vi "Set Panel Origin.vi"(8 "error in (no error)":errorcluster, 10 "origin":T1, 11 "reference":refnum<vi>) -> (0 "error out":errorcluster)   [LabVIEW 2019, in "UI Tools.lvlib"]
doc: "Set origin of the Panel."
uses:
  UI Tools.lvlib
  <vilib>/Utility/miscctls.llb/LVPointTypeDef.ctl
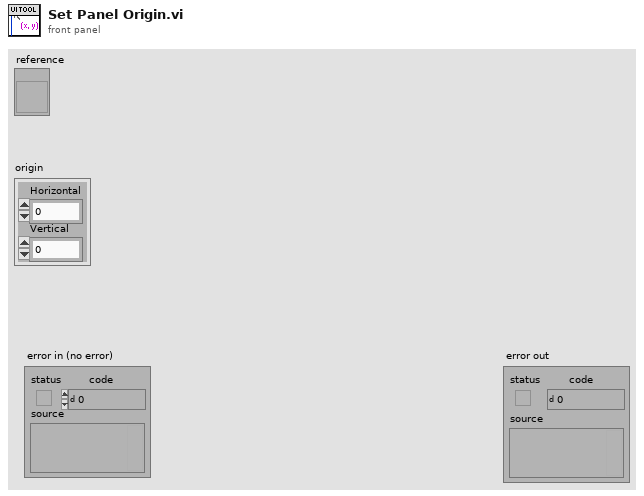
[diagram p1: front panel]
types:
  T1 = typedef "LVPointTypeDef.ctl" = cluster{"Horizontal":i16, "Vertical":i16}
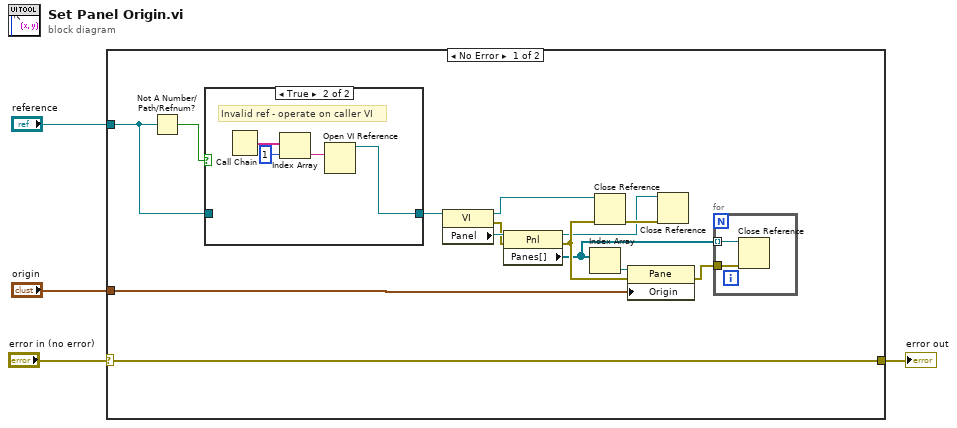
[diagram p0: block diagram]
diagram:
  n1 = case shown="No Error" "error in (no error)" {
    selector: "error in (no error)" -> [w18 w26]
    tunnel: [w18 w26] -> w3
    tunnel: "origin" -> [w5 _]
    tunnel: "reference" -> [w9 _]
    frame No Error {
      n2 = Not A Number/Path/Refnum?(number/path/refnum=w9) -> (NaN/Path/Refnum?=w10:bool)
      n3 = case shown="True" w10 {
        tunnel: [w19 w20] -> w8
        tunnel: w9 -> [w19 _]
        frame False {
        }
        frame True {
          # "Invalid ref - operate on caller VI"
          n4 = Call Chain() -> (call chain=w23:string[])
          n5 = Index Array(array=w23, index=1) -> (element=w21:string)
          n6 = Open VI Reference(vi path=w21) -> (vi reference=w20:refnum<vi>)  [unwired: 5 in, 1 out]
        }
      }
      n7 = property on="Property Node" class="VI"(reference=w8) -> (reference out=w12:refnum<vi>, error out=w15:errorcluster, "Panel"=w17:refnum<vi>)  [unwired: 1 in]
      n8 = property on="Property Node" class="Pnl"(reference=w17, error in=w15) -> (reference out=w6:refnum<vi>, error out=w13:errorcluster, "Panes[]"=w11:refnum<vi>[])
      n9 = Index Array(array=w11) -> (element=w16:refnum<vi>)  [unwired: 1 in]
      n10 = Close Reference(reference=w12, error in (no error)=w13) -> (error out=w7:errorcluster)
      n11 = property on="Property Node" class="Pane"(reference=w16, error in=w13, "Origin"=w5) -> (error out=w14:errorcluster)  [unwired: 1 out]
      n12 = Close Reference(reference=w6, error in (no error)=w7) -> ()  [unwired: 1 out]
      n13 = for {
        tunnel: w11 -> [w25] mode=indexing
        tunnel: w14 -> [w24]
        n14 = Close Reference(reference=w25, error in (no error)=w24) -> ()  [unwired: 1 out]
      }
    }
    frame Error {
    }
  }
  "error out" <- w3
